vi "Changing Panels Launcher.vi"   [LabVIEW 2020, in "2. Basic Panel Actors.lvlib"]
doc: "Launches the Chaning Panel Example.\n----\nCopyright: MGI 2017\nAuthor: Derek Trepanier"
uses:
  2. Basic Panel Actors.lvlib
  Changing Panels/Changing Panels.lvclass
  C:/Program Files/National Instruments/LabVIEW 2020/vi.lib/MGI/Panel Manager/Panel Actor/Panel Actor/Panel Actor.lvclass
  <vilib>/MGI/Panel Manager/Panel/Window Position/Reference Position/Alignment.ctl
  <vilib>/MGI/Panel Manager/Panel/Window Position/Reference Position/Horizontal Alignment.ctl
  <vilib>/MGI/Panel Manager/Panel/Window Position/Reference Position/Vertical Alignment.ctl
  <vilib>/MGI/Panel Manager/Panel/Window Position/Reference Position/Offset/Absolute Offset/No Offset.vi
  <vilib>/MGI/Panel Manager/Panel/Window Position/Reference Position/Offset/Absolute Offset/Absolute Offset.lvclass
  C:/Program Files/National Instruments/LabVIEW 2020/vi.lib/MGI/Panel Manager/Panel/Window Position/Reference Position/Offset/Offset.lvclass
  <vilib>/MGI/Panel Manager/Panel/Window Position/Reference Position/Ref Display/Ref Display.lvclass
  C:/Program Files/National Instruments/LabVIEW 2020/vi.lib/MGI/Panel Manager/Panel/Window Position/Window Position.lvclass
  <vilib>/MGI/Panel Manager/Panel/Window Position/Reference Position/Ref Display/Ref Display.vi
  <vilib>/MGI/Panel Manager/Panel Actor/Panel Actor/Launch Root Panel Window.vi
  <vilib>/MGI/Panel Manager/Panel Actor/Panel Actor/Panel Actor.lvclass
  <vilib>/MGI/Panel Manager/Panel/Panel.lvlib
  <vilib>/MGI/Panel Manager/Panel/Window Position/Reference Position/Reference Position.lvclass
  C:/Program Files/National Instruments/LabVIEW 2020/vi.lib/MGI/Panel Manager/Panel/Window Position/Reference Position/Offset/Absolute Offset/Absolute Offset.lvclass
  C:/Program Files/National Instruments/LabVIEW 2020/vi.lib/MGI/Panel Manager/Panel/Window Position/Reference Position/Reference Position.lvclass
  C:/Program Files/National Instruments/LabVIEW 2020/vi.lib/MGI/Panel Manager/Panel/Window Position/Reference Position/Ref Display/Ref Display.lvclass
  C:/Program Files/National Instruments/LabVIEW 2020/vi.lib/MGI/Monitored Actor/Monitored Actor/Monitored Actor/Monitored Actor.lvclass
  C:/Program Files/National Instruments/LabVIEW 2020/vi.lib/ActorFramework/Actor/Actor.lvclass
  C:/Program Files/National Instruments/LabVIEW 2020/examples/MGI/Panel Manager/Basic Panel Actors/Changing Panels/Changing Panels/Changing Panels.lvclass
panel:
  # "Run this VI to launch the Changing Panel example."
types:
  T1 = typedef "Panel.lvlib/Reference Position.lvclass/Alignment.ctl" = cluster{"Horizontal":T2, "Vertical":T3}
  T2 = typedef "Panel.lvlib/Reference Position.lvclass/Horizontal Alignment.ctl" = enum16{"Left", "Center", "Right"}
  T3 = typedef "Panel.lvlib/Reference Position.lvclass/Vertical Alignment.ctl" = enum16{"Top", "Center", "Bottom"}
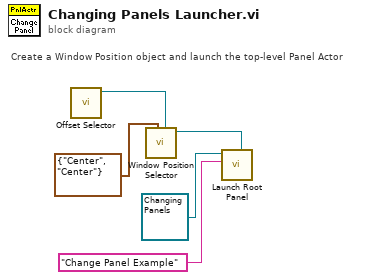
[diagram p0: block diagram]
diagram:
  # "Create a Window Position object and launch the top-level Panel Actor"
  n1 = call-poly <vilib>:"Offset Selector.vi"() -> ("Absolute Offset Out"=w2:refnum<class "Absolute Offset.lvclass">)  [unwired: 10 in, 1 out]
  n2 = call-poly <vilib>:"Window Position Selector.vi"("Offset"=w2, "Alignment"=T1 {"Horizontal"=enum."Center", "Vertical"=enum."Center"}) -> ("Ref Display out"=w3:refnum<class "Ref Display.lvclass">)  [unwired: 8 in, 1 out]
  n3 = call-poly <vilib>:"Launch Root Panel.vi"("Window Position (Maximize First Call)"=w3, "Title"="Change Panel Example", "Panel Actor in"=refnum<class "Changing Panels.lvclass"> refnum ("2. Basic Panel Actors.lvlib:Changing Panels.lvclass")) -> ()  [unwired: 7 in, 2 out]
